vi "Initialize.vi"(8 "error in (no error)":errorcluster) -> (0 "error out":errorcluster, 2 "queue out":refnum<queue>, 3 "Stream Download Controller out":refnum<class "Stream Download Controller.lvclass">)   [LabVIEW 2020, in "NI_SFTP.lvlib" / "Stream Download Controller.lvclass"]
uses:
  <vilib>/net/SFTP/API/Support/Download/Stream/Stream Download Controller.lvclass
  <vilib>/net/SFTP/API/Support/Download/Stream/Element.ctl
  <vilib>/net/SFTP/API/Support/Download/Stream/Stream Download Controller.lvclass/Stream Download Controller.ctl
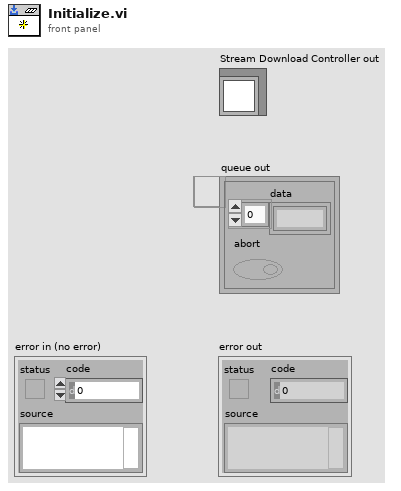
[diagram p1: front panel]
types:
  T1 = typedef "NI_SFTP.lvlib/Stream Download Controller.lvclass/Element.ctl" = cluster{"data":u8[], "abort":bool}
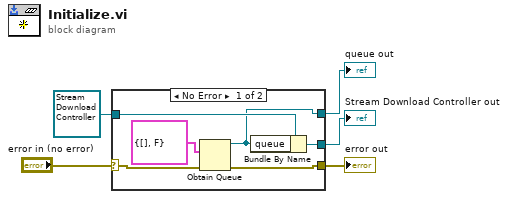
[diagram p0: block diagram]
diagram:
  n1 = case shown="No Error" "error in (no error)" {
    selector: "error in (no error)" -> [w9 w13]
    tunnel: [w8 w13] -> w4
    tunnel: [w11 w12] -> w2
    tunnel: refnum<class "Stream Download Controller.lvclass"> refnum ("Stream Download Controller in") -> [w10 w12]
    tunnel: [w7 _] -> w1
    frame No Error {
      n2 = Obtain Queue(element data type=T1 {"data"=[], "abort"=FALSE} ("element"), error in (no error)=w9) -> (queue out=w7:refnum<queue>, error out=w8:errorcluster)  [unwired: 3 in, 1 out]
      n3 = Bundle By Name(cluster=w10, "queue"=w7) -> (w11:refnum<class "Stream Download Controller.lvclass">)
    }
    frame Error {
    }
  }
  "error out" <- w4
  "Stream Download Controller out" <- w2
  "queue out" <- w1
